vi "Load Sound.vi"() -> (0 "error out":errorcluster, 3 "task ID out":T1 format="%.0x")   [LabVIEW 2019]
uses:
  <vilib>/sound2/lvsound2.llb/Sound Output Task ID.ctl
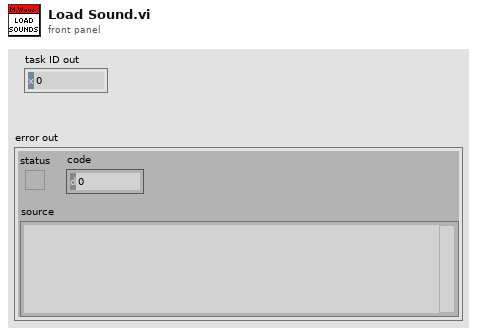
[diagram p1: front panel]
types:
  T1 = typedef "Sound Output Task ID.ctl" = u32
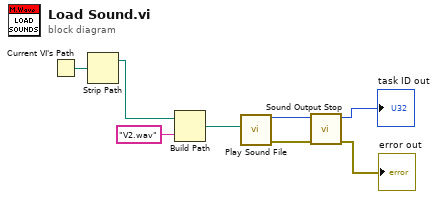
[diagram p0: block diagram]
diagram:
  n1 = Current VI's Path() -> (path=w8:path)
  n2 = Strip Path(path=w8) -> (stripped path=w1:path)  [unwired: 1 out]
  n3 = Build Path(base path=w1, name or relative path="V2.wav") -> (appended path=w6:path)
  n4 = call <vilib>:"Play Sound File.vi"("path"=w6) -> ("error out"=w5:errorcluster, "task ID"=w4:T1)  [unwired: 9 in]
  n5 = call <vilib>:"Sound Output Stop.vi"("error in (no error)"=w5, "task ID"=w4) -> ("error out"=→"error out":errorcluster, "task ID out"=→"task ID out":T1)  [unwired: 8 in]
